vi "CS POLARIS BME DG.ProcPeriodic.vi"(0 "i ref in":refnum<vi>, 3 "ms timeout (10000)":i32=10000, 5 "error in (no error)":errorcluster) -> (14 "i ref out":refnum<vi>, 17 "timed out":bool, 19 "error out":errorcluster)   [LabVIEW 2009, in "CS POLARIS BME DG.lvlib"]
doc: "This method serves to periodically do things like reading values from the HW. Methods that should be executed periodically should be called from THIS methode. Add code here."
uses:
  CS POLARIS BME DG.lvlib
  lib.lib/UtilityLib/UtilityLib.lvlib
  DG Classes/BME_DG_System/BME_DG_System.lvclass
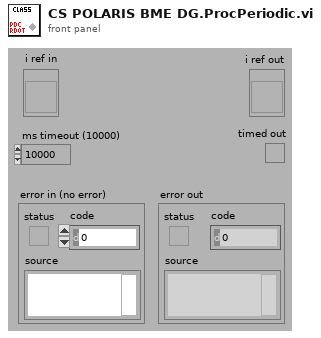
[diagram p1: front panel]
types:
  T1 = typedef "CS POLARIS BME DG.lvlib/CS POLARIS BME DG.i attribute.ctl" = cluster{"Numeric":dbl, "DG_System":refnum<queue>, "UpdateTasks":refnum<queue>}
  T2 = typedef "POLARIS BME DG.lvlib/Chnl Settings Complete.ctl" = cluster{"Channel Name":string, "ChnParameter":T3, "DelayFormula":string, "OutputModulo":i32, "Go and Done Signal":T4, "G08_Chnl_Settings":T6}
  T3 = typedef "POLARIS BME DG.lvlib/ChnlSettings.ctl" = cluster{" Delay (µs)":dbl, "On?":bool, "PositiveVoltage?":bool, "50OhmTerminated? ":bool, "25OhmOutput?":bool}
  T4 = typedef "POLARIS BME DG.lvlib/Go_Done_Chnl_Settings.ctl" = cluster{"Go Signal":T5, "Done Signal":u32}
  T5 = typedef "POLARIS BME DG.lvlib/GoSignalBits.ctl" = u32
  T6 = typedef "POLARIS BME DG.lvlib/SG08_Chnl_Settings.ctl" = cluster{"Pulse Width (µs)":dbl, "Output Offset":u32, "Disconnect (E,F)":bool, "Onto MsBus (E,F)":bool, "Input Positive (E,F)":bool}
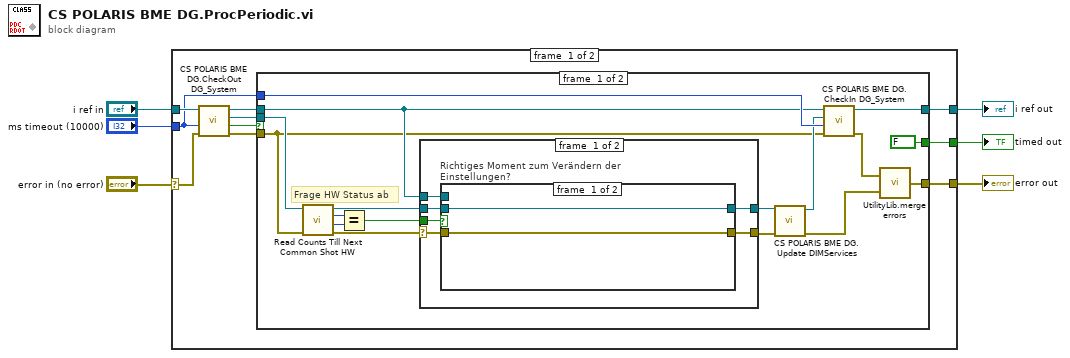
[diagram p0: block diagram]
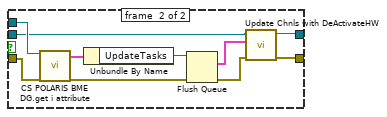
[diagram p2: hidden frame]
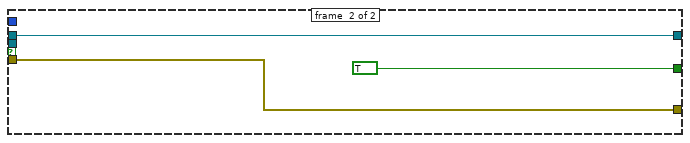
[diagram p4: hidden frame]
diagram:
  n1 = case shown="No Error" "error in (no error)" {
    selector: "error in (no error)" -> [w12 w57]
    tunnel: [w9 w57] -> w5
    tunnel: "i ref in" -> [w15 w58]
    tunnel: [w10 w58] -> w3
    tunnel: [w16 _] -> w2
    tunnel: "ms timeout (10000)" -> [w8 _]
    frame #0 {
      n2 = call "CS POLARIS BME DG.CheckOut DG_System.vi"("error IO"=w12, "timeout in ms (-1)"=w8, "i ref in"=w15) -> ("error out"=w13:errorcluster, "Q timed out"=w7:bool, "BME_DG_System out"=w14:refnum<class "BME_DG_System.lvclass">, "i ref out"=w11:refnum<vi>)  [unwired: 5 in]
      n3 = case shown="False" w7 {
        tunnel: [FALSE TRUE] -> w16
        tunnel: w14 -> [w18 _]
        tunnel: w13 -> [w17 w54]
        tunnel: w11 -> [w29 w55]
        tunnel: [w32 w55] -> w10
        tunnel: [w23 w54] -> w9
        tunnel: w8 -> [w30 _]
        frame #0 {
          # "Frage HW Status ab"
          n4 = call "Read Counts Till Next Common Shot HW.vi"("error in (no error)"=w17, "BME_DG_System in"=w18) -> ("error out"=w21:errorcluster, "LC Multiple"=w19:i64, "CountsRemains"=w20:i64, "BME_DG_System out"=w22:refnum<class "BME_DG_System.lvclass">)  [unwired: 5 in, 1 out]
          n5 = Equal?(x=w20, y=w19) -> (x = y?=w33:bool)
          n6 = case shown="No Error" w21 {
            selector: w21 -> [w38 w52]
            tunnel: w22 -> [w39 w53]
            tunnel: [w37 w52] -> w26
            tunnel: [w36 w53] -> w28
            tunnel: w33 -> [w35 _]
            tunnel: w29 -> [w34 _]
            frame #0 {
              n7 = case "Richtiges Moment zum Verändern der Einstellungen?" shown="True" w35 {
                tunnel: w39 -> [w41 w46]
                tunnel: w38 -> [w40 w50]
                tunnel: [w40 w44] -> w37
                tunnel: [w41 w45] -> w36
                tunnel: w34 -> [_ w51]
                frame #0 {
                }
                frame #1 {
                  n8 = call "CS POLARIS BME DG.get i attribute.vi"("i ref in"=w51, "error in (no error)"=w50) -> ("i attribute"=w48:T1, "error out"=w49:errorcluster)  [unwired: 15 in, 1 out]
                  n9 = Unbundle By Name(w48) -> ("UpdateTasks"=w47:refnum<queue>)
                  n10 = Flush Queue(queue=w47, error in (no error)=w49) -> (remaining elements=w42:T2[], error out=w43:errorcluster)  [unwired: 1 out]
                  n11 = call "Update Chnls with DeActivateHW.vi"("error in (no error)"=w43, "ChnlSettings"=w42, "BME_DG_System in"=w46) -> ("error out"=w44:errorcluster, "BME_DG_System out"=w45:refnum<class "BME_DG_System.lvclass">)  [unwired: 6 in, 1 out]
                }
              }
            }
            frame #1 {
            }
          }
          n12 = call "CS POLARIS BME DG.Update DIMServices.vi"("error in (no error)"=w26, "BME_DG_System in"=w28) -> ("error out"=w24:errorcluster, "BME_DG_System out"=w27:refnum<class "BME_DG_System.lvclass">)  [unwired: 8 in]
          n13 = call "CS POLARIS BME DG.CheckIn DG_System.vi"("error in"=w17, "timeout in ms (-1)"=w30, "BME_DG_System"=w27, "i ref in"=w29) -> ("error in"=w25:errorcluster, "i ref out"=w32:refnum<vi>)  [unwired: 5 in]
          n14 = call "UtilityLib.merge errors.vi"("error2 (no error)"=w24, "error1 (no error)"=w25) -> ("error out"=w23:errorcluster)
        }
        frame #1 {
        }
      }
    }
    frame #1 {
    }
  }
  "error out" <- w5
  "i ref out" <- w3
  "timed out" <- w2
